vi "Unit Vector PtByPt.vi"(0 "input data point":dbl format="%0.2f", 1 "sample length":i32=100, 2 "initialize":bool) -> (3 "Unit Vector":dbl[](array[numeric]), 4 "norm":dbl format="%0.2f", 5 "error":i32)   [LabVIEW 2020, in "NI_PtbyPt.lvlib"]
doc: "Finds the <B>norm</B> of the set of input data points specified by <B>sample length</B> and obtains its corresponding <B>Unit Vector</B> by normalizing the original set of input data points with its <B>norm</B>."
uses:
  NI_PtbyPt.lvlib
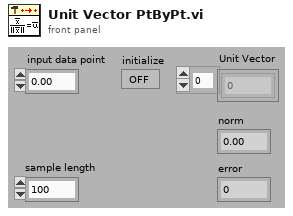
[diagram p1: front panel]
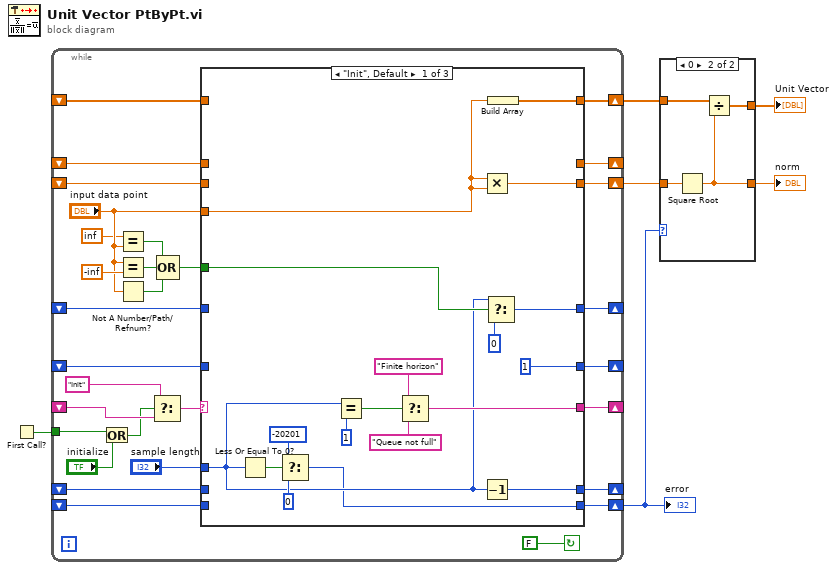
[diagram p0: block diagram]
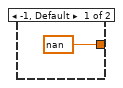
[diagram p2: hidden frame]
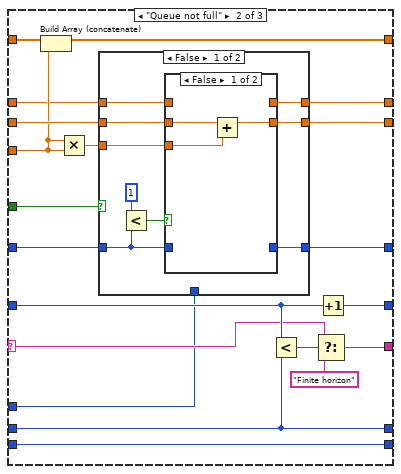
[diagram p3: hidden frame]
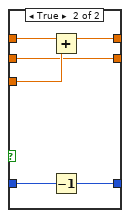
[diagram p4: hidden frame]
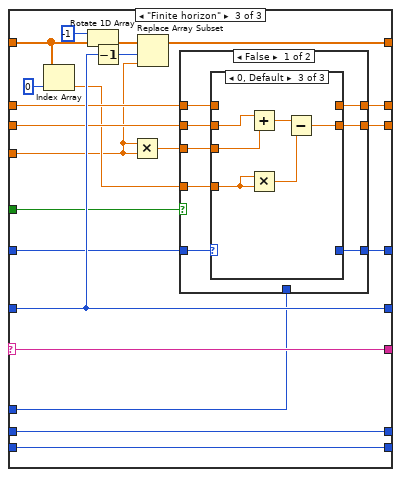
[diagram p6: hidden frame]
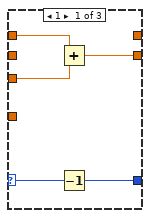
[diagram p7: hidden frame]
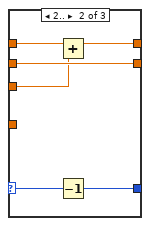
[diagram p8: hidden frame]
diagram:
  n1 = First Call?() -> (First Call?: T/F=w2:bool)
  n2 = while {
    tunnel: w2 -> [w22]
    shift-left: _ -> [w24]
    shift-right: [w25] -> _
    shift-left: _ -> [w27]
    shift-right: [w28] -> w4
    shift-left: _ -> [w30]
    shift-right: [w29] -> w6
    shift-left: _ -> [w32]
    shift-right: [w33] -> _
    shift-left: _ -> [w36]
    shift-right: [w31] -> _
    shift-right: [w12] -> _
    shift-left: _ -> [w10]
    shift-right: [w11] -> w1
    shift-left: _ -> [w7]
    shift-right: [w9] -> _
    shift-left: _ -> [w8]
    stop <- FALSE continue-if-true
    n3 = Or(x=w22, y="initialize") -> (x .or. y?=w20:bool)
    n4 = Equal?(x=inf, y="input data point") -> (x = y?=w17:bool)
    n5 = Equal?(x="input data point", y=-inf) -> (x = y?=w18:bool)
    n6 = Not A Number/Path/Refnum?(number/path/refnum="input data point") -> (NaN/Path/Refnum?=w16:bool)
    n7 = Select(t="Init", s=w20, f=w36) -> (s? t:f=w34:string)
    n8 = Compound Arithmetic op=OR(w17, w18, w16) -> (w13:bool)
    n9 = case shown="\"Init\", Default" w34 {
      selector: w34 -> [_ w70 w109]
      tunnel: "input data point" -> [w45 w64 w100]
      tunnel: [1 w62 w112] -> w33
      tunnel: w32 -> [_ w72 w112]
      tunnel: [w50 w68 w109] -> w31
      tunnel: w30 -> [_ w74 w110]
      tunnel: [w42 w73 w111] -> w29
      tunnel: "sample length" -> [w40 w56 w95]
      tunnel: [w44 w67 w107] -> w28
      tunnel: w27 -> [_ w66 w108]
      tunnel: [w43 w63 w106] -> w25
      tunnel: w24 -> [_ w63 w106]
      tunnel: w13 -> [w41 w61 w103]
      tunnel: [w39 w59 w98] -> w12
      tunnel: [w37 w55 w96] -> w11
      tunnel: w10 -> [_ w60 w104]
      tunnel: [_ w58 w97] -> w9
      tunnel: w8 -> [_ w57 w102]
      tunnel: w7 -> [_ w55 w96]
      frame "Init", Default {
        n10 = Less Or Equal To 0?(x=w40) -> (x <= 0?=w46:bool)
        n11 = Select(t=-20201, s=w46, f=0) -> (s? t:f=w37:i32)
        n12 = Equal?(x=w40, y=1) -> (x = y?=w52:bool)
        n13 = Select(t="Finite horizon", s=w52, f="Queue not full") -> (s? t:f=w50:string)
        n14 = Multiply(x=w45, y=w45) -> (x*y=w44:dbl)
        n15 = Decrement(x=w40) -> (x-1=w43:i32)
        n16 = Select(t=w40, s=w41, f=0) -> (s? t:f=w39:i32)
        n17 = Build Array(w45) -> (w42:dbl[])
      }
      frame "Queue not full" {
        n18 = Build Array (concatenate)(w74, w64) -> (w73:dbl[])
        n19 = Multiply(x=w64, y=w64) -> (x*y=w65:dbl)
        n20 = case shown="False" w61 {
          tunnel: [w83 w94] -> w67
          tunnel: w66 -> [w82 _]
          tunnel: w65 -> [w81 w94]
          tunnel: w60 -> [w78 _]
          tunnel: [w77 w93] -> w59
          tunnel: [w76 _] -> w58
          tunnel: w57 -> [w75 _]
          tunnel: w56 -> [_ w93]
          frame False {
            n21 = Less?(x=1, y=w78) -> (x < y?=w79:bool)
            n22 = case shown="False" w79 {
              tunnel: [w86 w87] -> w83
              tunnel: w82 -> [w85 w87]
              tunnel: w81 -> [w84 w88]
              tunnel: w78 -> [_ w92]
              tunnel: [_ w91] -> w77
              tunnel: [_ w90] -> w76
              tunnel: w75 -> [_ w89]
              frame False {
                n23 = Add(x=w85, y=w84) -> (x+y=w86:dbl)
              }
              frame True {
                n24 = Add(x=w89, y=w88) -> (x+y=w90:dbl)
                n25 = Decrement(x=w92) -> (x-1=w91:i32)
              }
            }
          }
          frame True {
          }
        }
        n26 = Less?(x=w72, y=w63) -> (x < y?=w71:bool)
        n27 = Select(t=w70, s=w71, f="Finite horizon") -> (s? t:f=w68:string)
        n28 = Increment(x=w72) -> (x+1=w62:i32)
      }
      frame "Finite horizon" {
        n29 = Index Array(array=w110, index=0 ("Index")) -> (element=w101:dbl)
        n30 = Rotate 1D Array(1:w110, 2:i16 -1 ("n")) -> (0:w113:dbl[])
        n31 = Decrement(x=w112) -> (x-1=w105:i32)
        n32 = Multiply(x=w100, y=w100) -> (x*y=w99:dbl)
        n33 = Replace Array Subset(array=w113, new element=w100, index=w105) -> (w111:dbl[])
        n34 = case shown="False" w103 {
          tunnel: w108 -> [w123 _]
          tunnel: [w122 w142] -> w107
          tunnel: w99 -> [w121 w142]
          tunnel: w101 -> [w120 _]
          tunnel: w104 -> [w119 _]
          tunnel: w102 -> [w118 _]
          tunnel: [w117 w141] -> w98
          tunnel: [w116 _] -> w97
          tunnel: w95 -> [_ w141]
          frame False {
            n35 = case shown="0, Default" w119 {
              selector: w119 -> [w125 w134 _]
              tunnel: w123 -> [_ w132 w140]
              tunnel: [w126 w132 w138] -> w122
              tunnel: w121 -> [w128 w129 w135]
              tunnel: w120 -> [_ _ w137]
              tunnel: w118 -> [w127 w130 _]
              tunnel: [w124 w133 _] -> w117
              tunnel: [_ w131 _] -> w116
              frame 1 {
                n36 = Add(x=w127, y=w128) -> (x+y=w126:dbl)
                n37 = Decrement(x=w125) -> (x-1=w124:i32)
              }
              frame 2.. {
                n38 = Add(x=w130, y=w129) -> (x+y=w131:dbl)
                n39 = Decrement(x=w134) -> (x-1=w133:i32)
              }
              frame 0, Default {
                n40 = Add(x=w140, y=w135) -> (x+y=w139:dbl)
                n41 = Multiply(x=w137, y=w137) -> (x*y=w136:dbl)
                n42 = Subtract(x=w139, y=w136) -> (x-y=w138:dbl)
              }
            }
          }
          frame True {
          }
        }
      }
    }
  }
  "error" <- w1
  n43 = case shown="0" w1 {
    tunnel: w6 -> [_ w147]
    tunnel: [_ w146] -> w5
    tunnel: w4 -> [_ w145]
    tunnel: [nan w144] -> w3
    frame -1, Default {
    }
    frame 0 {
      n44 = Square Root(x=w145) -> (sqrt(x)=w144:dbl)
      n45 = Divide(x=w147, y=w144) -> (x/y=w146:dbl[])
    }
  }
  "Unit Vector" <- w5
  "norm" <- w3
